vi "CLD 2 Elapsed Time Express FGV Self Solution.vi"(7 "Express Timer FGV Enum":enum16{"Reset", "Read Status", "Set Auto Reset"}(ring), 8 "error in (no error)":errorcluster, 9 "Auto Reset (F)":bool, 11 "Time Target (s)":dbl=7.0) -> (0 "error out":errorcluster, 2 "Elapsed Time (s)":dbl, 3 "Time Has Elapsed":bool)   [LabVIEW 2015]
doc: "CLD 2 Exercise"
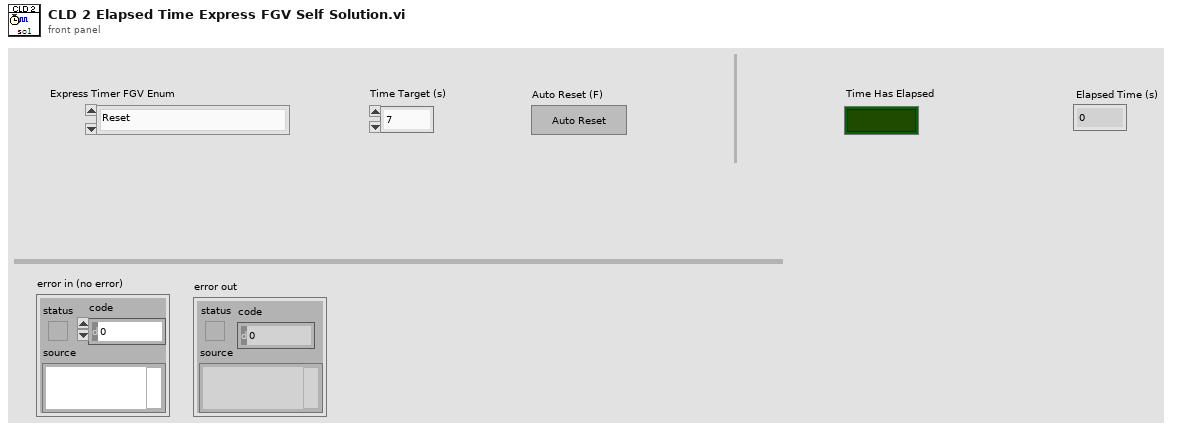
[diagram p1: front panel]
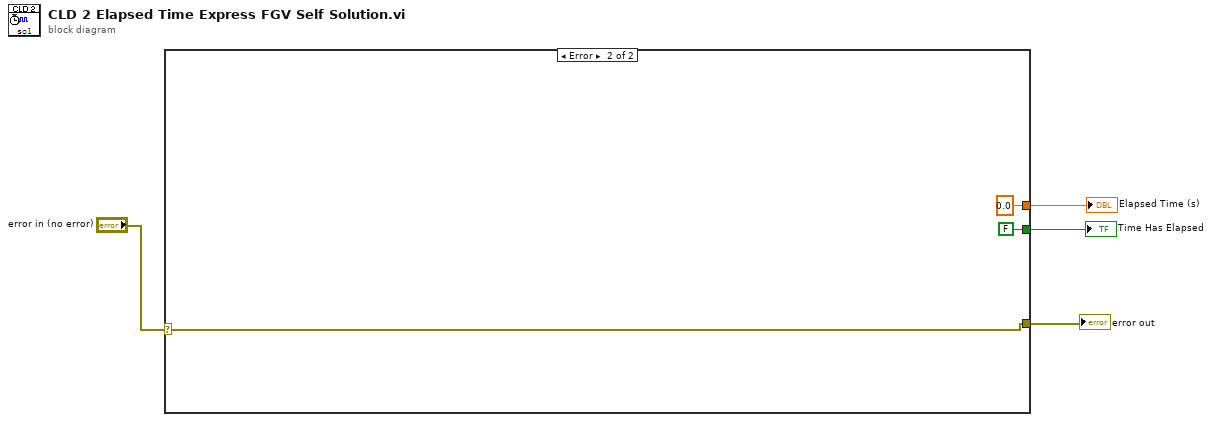
[diagram p0: block diagram]
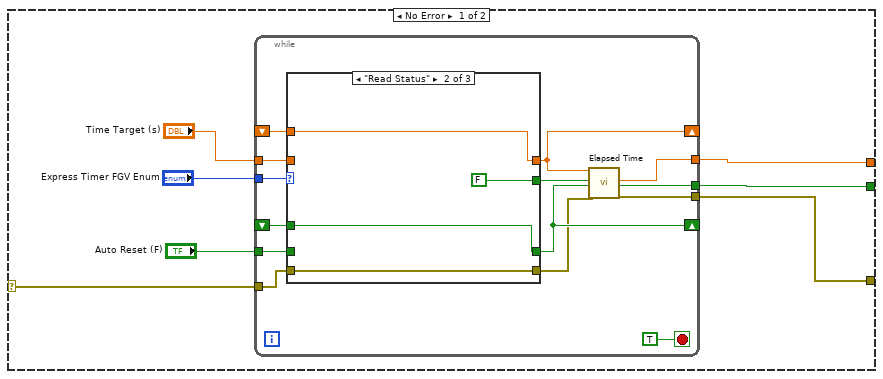
[diagram p2: hidden frame]
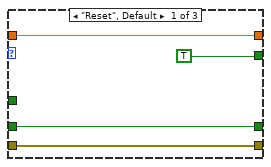
[diagram p3: hidden frame]
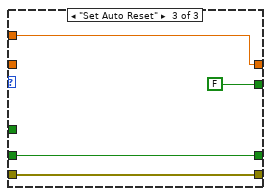
[diagram p4: hidden frame]
diagram:
  n1 = case shown="Error" "error in (no error)" {
    selector: "error in (no error)" -> [w8 w40]
    tunnel: [w7 w40] -> w3
    tunnel: [w6 0.0 ("Elapsed Time (s)")] -> w2
    tunnel: [w5 FALSE ("Time has Elapsed")] -> w1
    frame No Error {
      n2 = while {
        tunnel: "Express Timer FGV Enum" -> [w24]
        tunnel: [w22] -> w5
        shift-right: [w20] -> _
        shift-left: _ -> [w19]
        tunnel: "Time Target (s)" -> [w21]
        shift-right: [w16] -> _
        shift-left: _ -> [w18]
        tunnel: "Auto Reset (F)" -> [w17]
        tunnel: [w15] -> w6
        tunnel: w8 -> [w14]
        tunnel: [w12] -> w7
        stop <- TRUE stop-if-true
        n3 = case shown="\"Read Status\"" w24 {
          tunnel: [TRUE FALSE FALSE] -> w23
          tunnel: w21 -> [w28 _ _]
          tunnel: [w28 w32 w36] -> w20
          tunnel: w19 -> [_ w32 w36]
          tunnel: w18 -> [_ w31 _]
          tunnel: [w27 w31 w35] -> w16
          tunnel: w17 -> [w27 _ w35]
          tunnel: w14 -> [w26 w30 w34]
          tunnel: [w26 w30 w34] -> w13
          frame "Reset", Default {
          }
          frame "Read Status" {
          }
          frame "Set Auto Reset" {
          }
        }
        n4 = call "Elapsed Time"("Time Target (s)"=w20, "Reset"=w23, "Auto Reset"=w16, "error in (no error)"=w13) -> ("Elapsed Time (s)"=w15:dbl, "Time has Elapsed"=w22:bool, "error out"=w12:errorcluster)  [unwired: 8 in, 5 out]
      }
    }
    frame Error {
    }
  }
  "error out" <- w3
  "Elapsed Time (s)" <- w2
  "Time Has Elapsed" <- w1
